vi "簇.vi"() -> ()   [LabVIEW 2020]
panel:
  out "报警指示":bool
  in  "报警值":dbl
  out "温度":dbl
  out "数值 4":dbl
  out "簇 5":cluster{"学号":dbl, "名字":string}
  out "字符串 2":string
  out "数值 2":dbl
  out "字符串":string
  out "数值":dbl
  out "簇 4":cluster{"学号":dbl, "布尔":bool, "名字":string}
  in  "簇 3":cluster{"学号":dbl, "布尔":bool, "名字":string}
  out "簇 2":cluster{"学号":dbl, "布尔":bool, "名字":string}
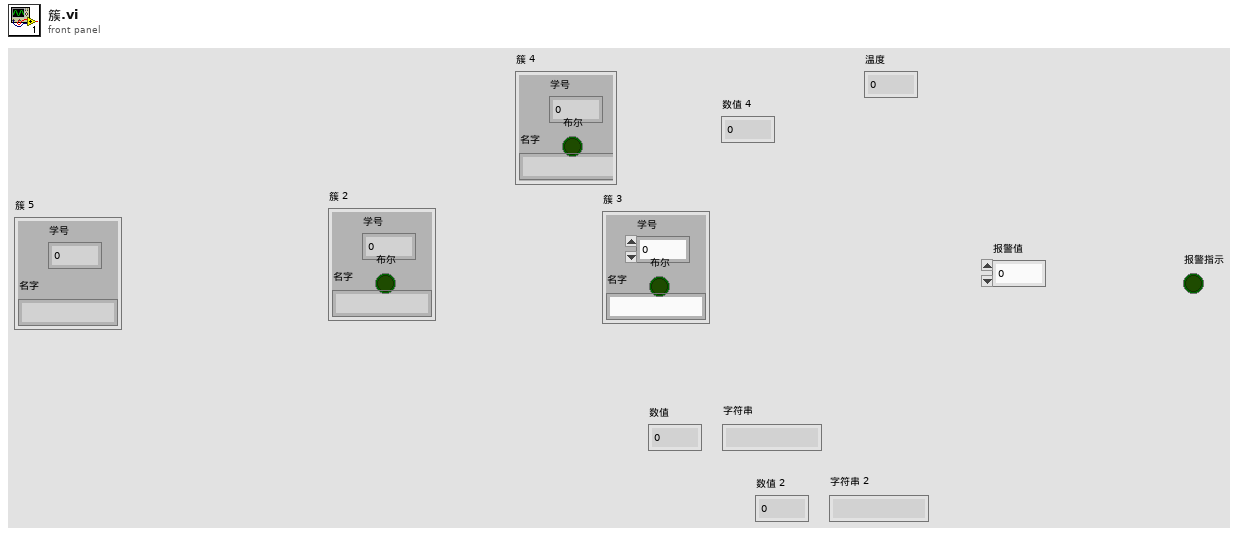
[diagram p1: front panel]
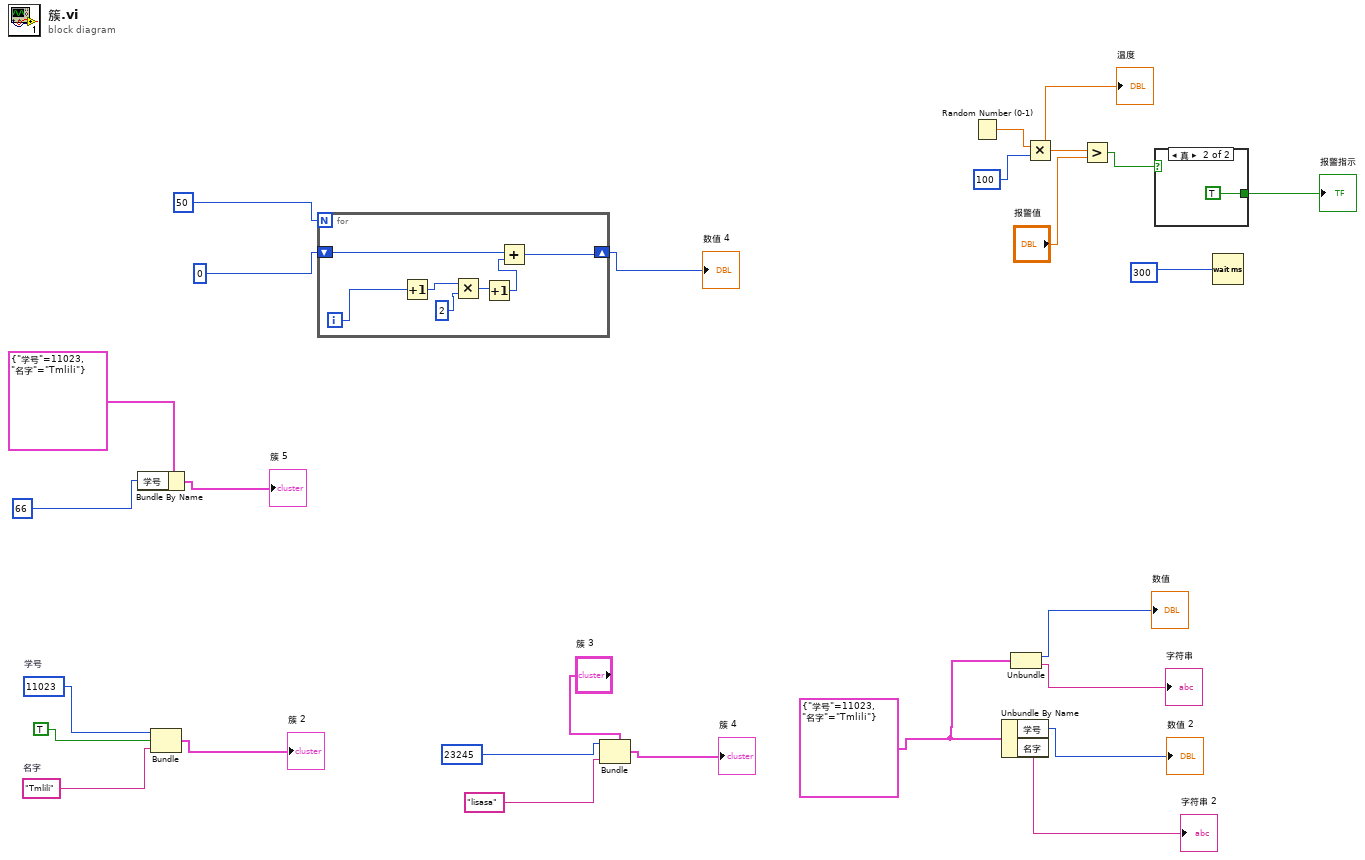
[diagram p0: block diagram]
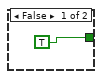
[diagram p2: hidden frame]
diagram:
  w18 = cluster{"学号":i32, "名字":string} {"学号"=11023, "名字"="Tmlili"}
  w24 = "Tmlili"  # 名字
  w26 = 11023  # 学号
  n1 = Bundle By Name(cluster=cluster{"学号":i32, "名字":string} {"学号"=11023, "名字"="Tmlili"}, "学号"=66) -> (→"簇 5":cluster{"学号":i32, "名字":string})
  n2 = Bundle("学号"=w26, TRUE, "名字"=w24) -> (→"簇 2":cluster{"学号":i32, bool, "名字":string})  [unwired: 1 in]
  n3 = for {
    N: 50 -> [_]
    shift-right: [w31] -> w8
    shift-left: 0 -> [w32]
    i -> [w33]
    n4 = Increment(x=w33) -> (x+1=w30:i32)
    n5 = Multiply(x=w30, y=2) -> (x*y=w28:i32)
    n6 = Increment(x=w28) -> (x+1=w27:i32)
    n7 = Add(x=w32, y=w27) -> (x+y=w31:i32)
  }
  "数值 4" <- w8
  n8 = Bundle(cluster="簇 3", "学号"=23245, "名字"="lisasa") -> (→"簇 4":cluster{"学号":dbl, "布尔":bool, "名字":string})  [unwired: 1 in]
  n9 = Random Number (0-1)() -> (number: 0 to 1=w6:dbl)
  n10 = Unbundle By Name(w18) -> ("学号"=→"数值 2":i32, "名字"=→"字符串 2":string)
  n11 = Unbundle(w18) -> ("学号"=→"数值":i32, "名字"=→"字符串":string)
  n12 = Multiply(x=w6, y=100) -> (x*y=w4:dbl)
  "温度" <- w4
  n13 = Greater?(x=w4, y="报警值") -> (0:w3:bool)
  n14 = case shown="真" w3 {
    tunnel: [TRUE TRUE] -> w1
    frame False {
    }
    frame True {
    }
  }
  "报警指示" <- w1
  n15 = Wait (ms)(milliseconds to wait=300) -> ()  [unwired: 1 out]
